vi "DynamixelEdit_ID_Helper.vi"() -> ()   [LabVIEW 2013]
uses:
  <instrlib>/Dynamixel Motor/Dynamixel Motor.lvlib
panel:
  in  "New ID":u8
  in  "Current ID":u8
  out "Motors IDs Found":u8[](array[numeric])
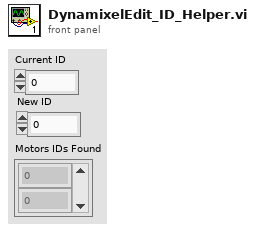
[diagram p1: front panel]
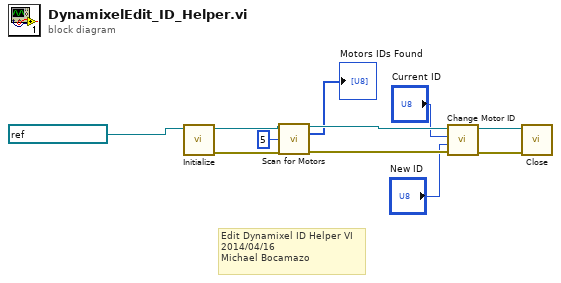
[diagram p0: block diagram]
diagram:
  # "Edit Dynamixel ID Helper VI\n2014/04/16 \nMichael Bocamazo"
  n1 = call <instrlib>:"Initialize.vi"("VISA resource name"=refnum<visa-resource-name> "ASRL3::INSTR") -> ("error out"=w8:errorcluster, "VISA resource name out"=w9:refnum<visa-resource-name>)  [unwired: 9 in]
  n2 = call <instrlib>:"Scan for Motors.vi"("VISA resource name"=w9, "Ending ID (253)"=u8 5, "error in (no error)"=w8) -> ("VISA resource name out"=w7:refnum<visa-resource-name>, "Motors IDs Found"=→"Motors IDs Found":u8[], "error out"=w4:errorcluster)  [unwired: 10 in]
  n3 = call <instrlib>:"Change Motor ID.vi"("error in (no error)"=w4, "New ID"="New ID", "Current ID"="Current ID", "VISA resource name"=w7) -> ("error out"=w5:errorcluster, "VISA Resource Out"=w6:refnum<visa-resource-name>)  [unwired: 6 in]
  n4 = call <instrlib>:"Close.vi"("error in (no error)"=w5, "VISA resource name"=w6) -> ()  [unwired: 9 in, 1 out]
